vi "Convert Raw Frame to Data.vi"(7 "Database alias":string="Database", 8 "error in (no error)":errorcluster, 11 "Raw Frames":T2[](array[typedef])=[{"timestamp"=timestamp(0 s since 1904-01-01), "payload"=[243, 96, 137, 220, 5, 1, 0, 32], "identifier"=1281, "type"=0, "extended?"=FALSE, "echo?"=FALSE}] {"payload" format="%x"; "timestamp" format="%<%.7X\n%x>T"; "type" items=["CAN Data"=0, "CAN Remote"=1, "CAN Bus Error"=2, "CAN 2.0 Data"=8, "CAN FD Data"=16, "CAN FD+BRS Data"=24, "J1939 Data"=192, "Delay"=224, "Log Trigger"=225, "Start Trigger"=226]; "identifier" format="%x"}) -> (0 "error out":errorcluster, 3 "Frame Data":T1[](array[typedef]) {"Raw Frame"."payload" format="%x"; "Raw Frame"."timestamp" format="%<%.7X\n%x>T"; "Raw Frame"."type" items=["CAN Data"=0, "CAN Remote"=1, "CAN Bus Error"=2, "CAN 2.0 Data"=8, "CAN FD Data"=16, "CAN FD+BRS Data"=24, "J1939 Data"=192, "Delay"=224, "Log Trigger"=225, "Start Trigger"=226]; "Raw Frame"."identifier" format="%x"})   [LabVIEW 2021]
uses:
  <vilib>/xnet/xnet.llb/XNET Frame CAN.ctl
  <vilib>/xnet/xnet.llb/XNET Frame Type CAN.ctl
  controls/Frame Data.ctl
  controls/Signal Data.ctl
  <vilib>/xnet/xnet.llb/XNET Create Session (Conversion).vi
  <vilib>/xnet/xnet.llb/XNET Convert (Frame CAN to Signal).vi
  <resource>/objmgr/xnet.rc
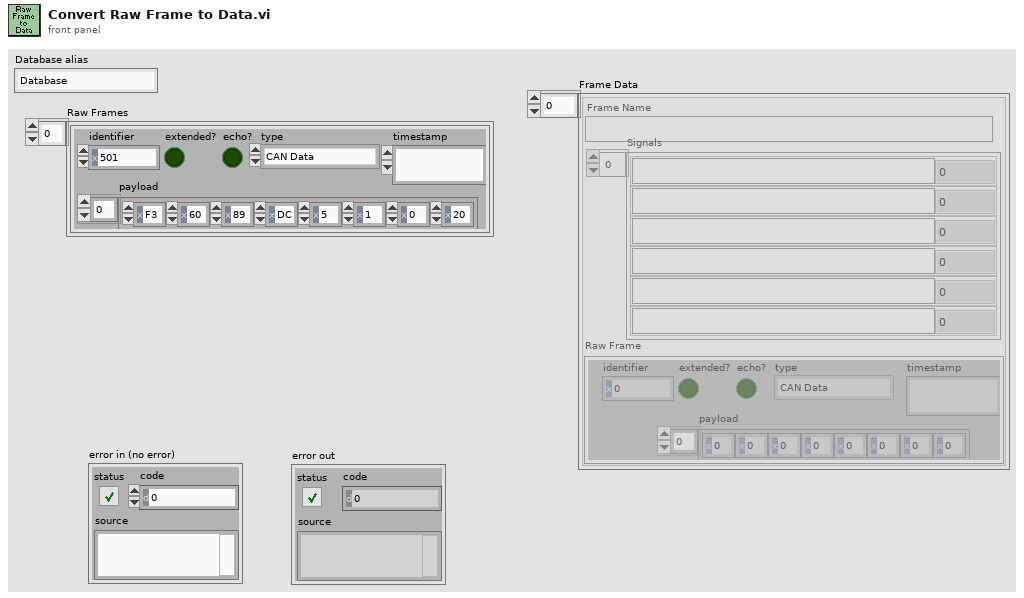
[diagram p1: front panel]
types:
  T1 = typedef "Frame Data.ctl" = cluster{"Raw Frame":T2, "Frame Name":refnum<k21>, "Signals":T4[]}
  T2 = typedef "XNET Frame CAN.ctl" = cluster{"timestamp":timestamp, "payload":u8[], "identifier":u32, "type":T3, "extended?":bool, "echo?":bool}
  T3 = typedef "XNET Frame Type CAN.ctl" = u8
  T4 = typedef "Signal Data.ctl" = cluster{"XNET Signal":refnum<k21>, "Data":dbl}
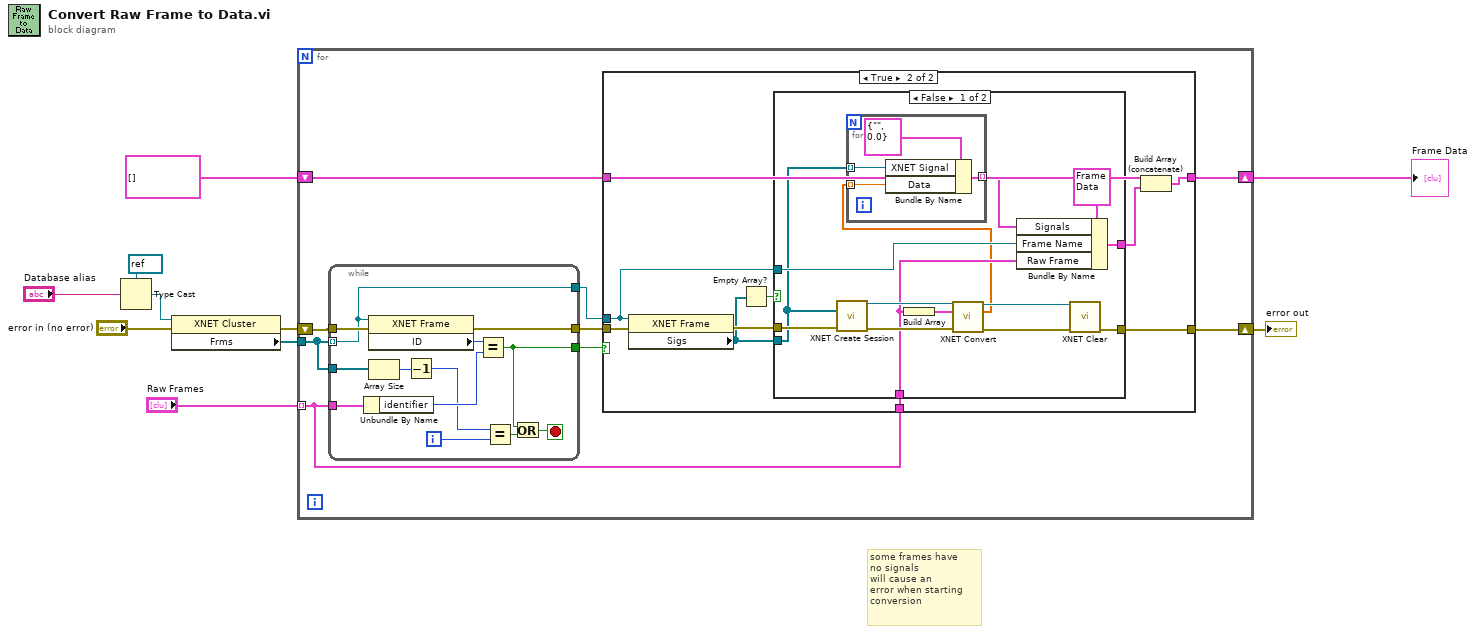
[diagram p0: block diagram]
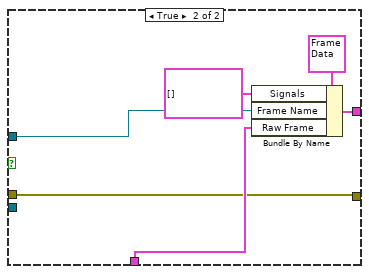
[diagram p3: hidden frame]
diagram:
  # "some frames have\nno signals\nwill cause an \nerror when starting\nconversion"
  n1 = Type Cast(type=refnum<k21> refnum ("cluster (:memory:)"), x="Database alias") -> (*(type *) &x=w2:refnum<k21>)
  n2 = property class="XNET Cluster"(reference=w2, error in="error in (no error)") -> (error out=w7:errorcluster, "Frms"=w10:refnum<k21>[])  [unwired: 1 out]
  n3 = for {
    tunnel: w10 -> [w19]
    tunnel: "Raw Frames" -> [w16] mode=indexing
    shift-right: [w13] -> w1
    shift-left: T1[] [] ("Array") -> [w14]
    shift-right: [w12] -> w6
    shift-left: w7 -> [w11]
    n4 = while {
      tunnel: w19 -> [w56] mode=indexing
      tunnel: w11 -> [w68]
      tunnel: w16 -> [w66]
      tunnel: w19 -> [w63]
      tunnel: [w56] -> w18
      tunnel: [w60] -> w15
      tunnel: [w59] -> w17
      i -> [w57]
      stop <- w64 stop-if-true
      n5 = Unbundle By Name(w66) -> ("identifier"=w65:u32)
      n6 = property class="XNET Frame"(reference=w56, error in=w68) -> (error out=w59:errorcluster, "ID"=w67:u32)  [unwired: 1 out]
      n7 = Array Size(array=w63) -> (size(s)=w62:i32)
      n8 = Decrement(x=w62) -> (x-1=w58:i32)
      n9 = Equal?(x=w67, y=w65) -> (x = y?=w60:bool)
      n10 = Equal?(x=w58, y=w57) -> (x = y?=w61:bool)
      n11 = Or(x=w60, y=w61) -> (x .or. y?=w64:bool)
    }
    n12 = case shown="True" w15 {
      tunnel: w18 -> [_ w24]
      tunnel: w17 -> [w20 w31]
      tunnel: w16 -> [_ w29]
      tunnel: w14 -> [w21 w28]
      tunnel: [w21 w26] -> w13
      tunnel: [w20 w25] -> w12
      frame False {
      }
      frame True {
        n13 = property class="XNET Frame"(reference=w24, error in=w31) -> (error out=w30:errorcluster, "Sigs"=w23:refnum<k21>[])  [unwired: 1 out]
        n14 = Empty Array?(array=w23) -> (empty?=w22:bool)
        n15 = case shown="False" w22 {
          tunnel: w30 -> [w44 w50]
          tunnel: w23 -> [w34 _]
          tunnel: w29 -> [w40 w51]
          tunnel: [w39 w54] -> w27
          tunnel: [w36 w50] -> w25
          tunnel: w24 -> [w35 w53]
          frame False {
            n16 = call-poly <vilib>:"XNET Create Session.vi"("signal list"=w34, "error in (no error)"=w44) -> ("session out"=w43:refnum<k21>, "error out"=w41:errorcluster)  [unwired: 12 in]
            n17 = Build Array(w40) -> (w42:T2[])
            n18 = call-poly <vilib>:"XNET Convert.vi"("session in"=w43, "frame data"=w42, "error in (no error)"=w41) -> ("session out"=w38:refnum<k21>, "signal data"=w33:dbl[], "error out"=w37:errorcluster)  [unwired: 10 in]
            n19 = for {
              tunnel: w34 -> [w48] mode=indexing
              tunnel: w33 -> [w47] mode=indexing
              tunnel: [w46] -> w32 mode=indexing
              n20 = Bundle By Name(cluster=T4 {"XNET Signal"="", "Data"=0.0} ("Signal"), "XNET Signal"=w48, "Data"=w47) -> (w46:T4)
            }
            n21 = Bundle By Name(cluster=T1 {"Raw Frame"={"timestamp"=timestamp(0 s since 1904-01-01), "payload"=[], "identifier"=0, "type"=0, "extended?"=FALSE, "echo?"=FALSE}, "Frame Name"="", "Signals"=[]} ("Frame Data"), "Signals"=w32, "Frame Name"=w35, "Raw Frame"=w40) -> (w39:T1)
            n22 = call <vilib>:"XNET Clear.vi"("session in"=w38, "error in (no error)"=w37) -> ("error out"=w36:errorcluster)  [unwired: 13 in]
          }
          frame True {
            n23 = Bundle By Name(cluster=T1 {"Raw Frame"={"timestamp"=timestamp(0 s since 1904-01-01), "payload"=[], "identifier"=0, "type"=0, "extended?"=FALSE, "echo?"=FALSE}, "Frame Name"="", "Signals"=[]} ("Frame Data"), "Signals"=T4[] [], "Frame Name"=w53, "Raw Frame"=w51) -> (w54:T1)
          }
        }
        n24 = Build Array (concatenate)(w28, w27) -> (w26:T1[])
      }
    }
  }
  "error out" <- w6
  "Frame Data" <- w1
